vi "TDM Registry.vi"(8 "Details":T2, 9 "Delivery Notifier":refnum<notifier>, 10 "TDM ID":string, 11 "Action":T1) -> (0 "Details out":T2, 1 "Delivery Notifier":refnum<notifier>, 2 "TDM ID out":string, 3 "Found":bool, 4 "TDM Alias Out":string)   [LabVIEW 2020, in "Actor Framework.lvlib"]
uses:
  Actor Framework.lvlib
  Time-Delayed Send Message/Time-Delay Override Options.ctl
  TDM Registration Mode.ctl
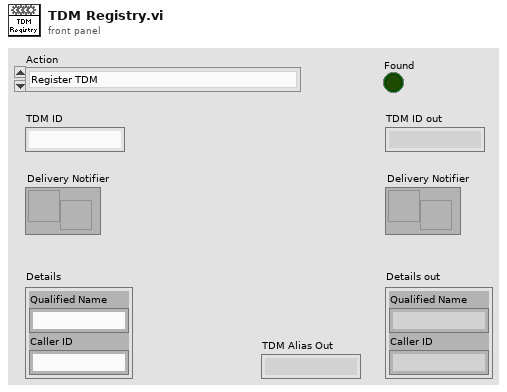
[diagram p1: front panel]
types:
  T1 = typedef "Actor Framework.lvlib/TDM Registration Mode.ctl" = enum16{"Register TDM", "Get ID", "Get Notifier", "Deregister TDM"}
  T2 = cluster{"Qualified Name":string, "Caller ID":string}
  T3 = cluster{"Enqueuers":refnum<notifier>[], "IDs":string[], "Details":cluster{"Qualified Name":string, "Caller ID":string}[]}
  T4 = cluster{"Qualified Name":string, "Caller ID":string}[]
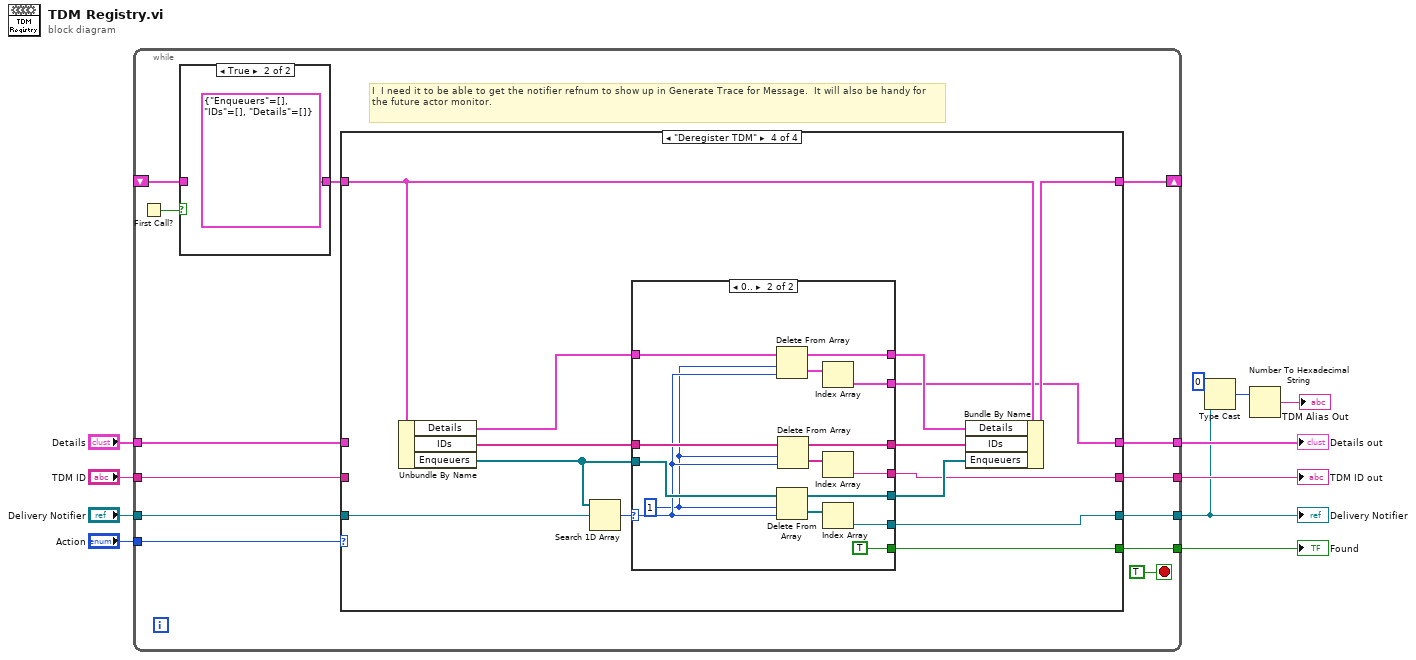
[diagram p0: block diagram]
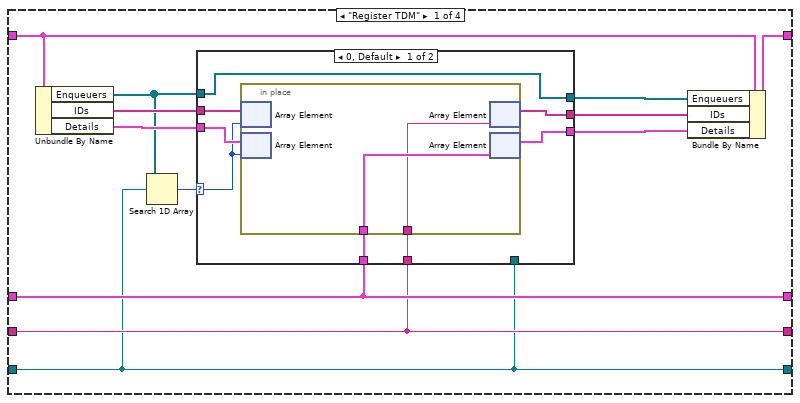
[diagram p3: hidden frame]
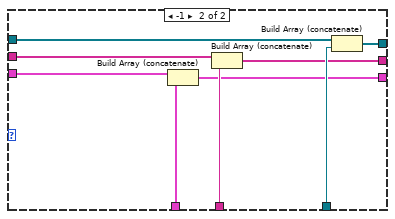
[diagram p4: hidden frame]
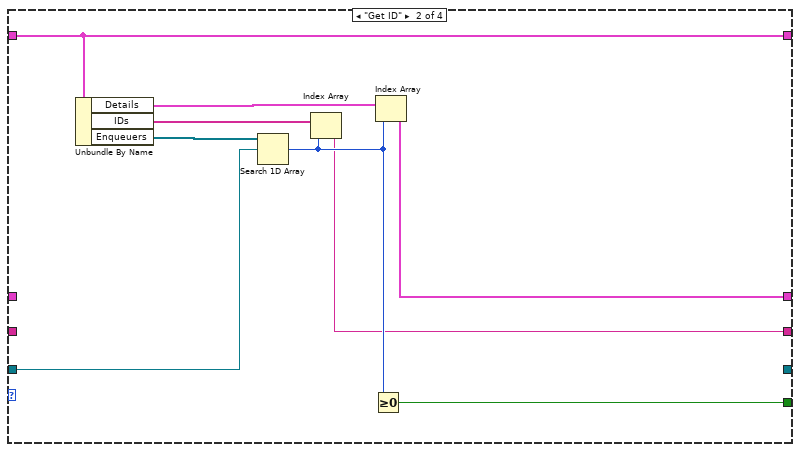
[diagram p5: hidden frame]
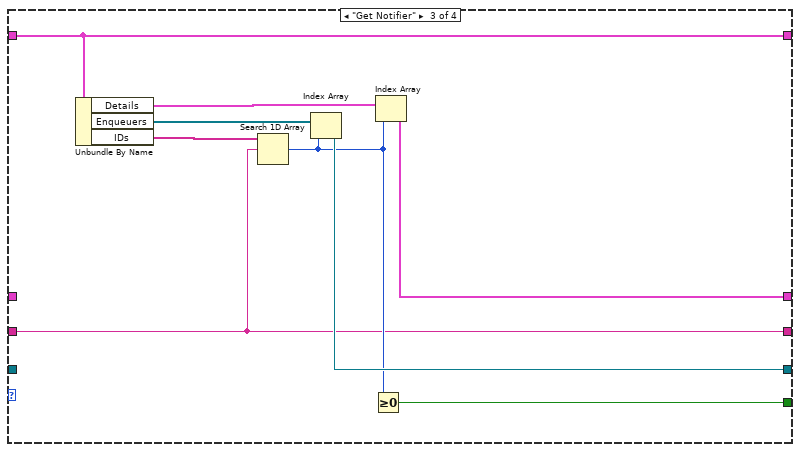
[diagram p6: hidden frame]
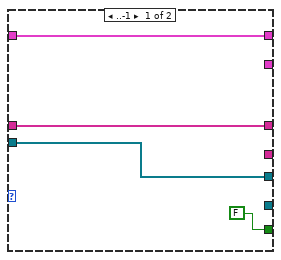
[diagram p7: hidden frame]
diagram:
  n1 = while {
    tunnel: "Action" -> [w24]
    shift-right: [w23] -> _
    shift-left: _ -> [w13]
    tunnel: "TDM ID" -> [w22]
    tunnel: "Delivery Notifier" -> [w21]
    tunnel: "Details" -> [w20]
    tunnel: [w15] -> w5
    tunnel: [w18] -> w7
    tunnel: [w17] -> w6
    tunnel: [w16] -> w2
    stop <- TRUE stop-if-true
    # "I  I need it to be able to get the notifier refnum to show up in Generate Trace for Message.  It will also be handy for the future actor monitor."
    n2 = First Call?() -> (First Call?: T/F=w12:bool)
    n3 = case shown="True" w12 {
      tunnel: [w25 T3 {"Enqueuers"=[], "IDs"=[], "Details"=[]}] -> w14
      tunnel: w13 -> [w25 _]
      frame False {
      }
      frame True {
      }
    }
    n4 = case shown="\"Deregister TDM\"" w24 {
      tunnel: w14 -> [w32 w62 w72 w84]
      tunnel: [w38 w62 w72 w79] -> w23
      tunnel: w22 -> [w28 _ w67 _]
      tunnel: w21 -> [w27 w65 _ w85]
      tunnel: w20 -> [w29 _ _ _]
      tunnel: [w28 w58 w67 w77] -> w15
      tunnel: [w29 w60 w69 w76] -> w18
      tunnel: [_ w61 w71 w80] -> w17
      tunnel: [w27 _ w70 w78] -> w16
      frame "Register TDM" {
        n5 = Unbundle By Name(w32) -> ("Enqueuers"=w31:refnum<notifier>[], "IDs"=w35:string[], "Details"=w34:T4)
        n6 = Search 1D Array(1D array=w31, element=w27) -> (index of element=w30:i32)  [unwired: 1 in]
        n7 = case shown="0, Default" w30 {
          selector: w30 -> [w39 _]
          tunnel: w28 -> [w44 w57]
          tunnel: w27 -> [_ w56]
          tunnel: w29 -> [w45 w55]
          tunnel: w31 -> [w46 w54]
          tunnel: [w46 w53] -> w37
          tunnel: [w41 w52] -> w36
          tunnel: w35 -> [w43 w51]
          tunnel: w34 -> [w42 w50]
          tunnel: [w40 w49] -> w33
          frame 0, Default {
            n8 = in-place {
              in-place-border: w45 -> [w48]
              in-place-border: w44 -> [w47]
              n9 = in-place-array #1(w43, w39) -> ()  [unwired: 1 out]
              n10 = in-place-array #2(w42, w39) -> ()  [unwired: 1 out]
              n11 = in-place-array #1(w47) -> (w41:string[])  [unwired: 1 out]
              n12 = in-place-array #2(w48) -> (w40:T4)  [unwired: 1 out]
            }
          }
          frame -1 {
            n13 = Build Array (concatenate)(w50, w55) -> (w49:T4)
            n14 = Build Array (concatenate)(w51, w57) -> (w52:string[])
            n15 = Build Array (concatenate)(w54, w56) -> (w53:refnum<notifier>[])
          }
        }
        n16 = Bundle By Name(cluster=w32, "Enqueuers"=w37, "IDs"=w36, "Details"=w33) -> (w38:T3)
      }
      frame "Get ID" {
        n17 = Unbundle By Name(w62) -> ("Details"=w64:T4, "IDs"=w63:string[], "Enqueuers"=w66:refnum<notifier>[])
        n18 = Search 1D Array(1D array=w66, element=w65) -> (index of element=w59:i32)  [unwired: 1 in]
        n19 = Index Array(array=w63, index=w59) -> (element=w58:string)
        n20 = Greater Or Equal To 0?(x=w59) -> (x >= 0?=w61:bool)
        n21 = Index Array(array=w64, index=w59) -> (element=w60:T2)
      }
      frame "Get Notifier" {
        n22 = Unbundle By Name(w72) -> ("Details"=w74:T4, "Enqueuers"=w73:refnum<notifier>[], "IDs"=w75:string[])
        n23 = Search 1D Array(1D array=w75, element=w67) -> (index of element=w68:i32)  [unwired: 1 in]
        n24 = Index Array(array=w73, index=w68) -> (element=w70:refnum<notifier>)
        n25 = Greater Or Equal To 0?(x=w68) -> (x >= 0?=w71:bool)
        n26 = Index Array(array=w74, index=w68) -> (element=w69:T2)
      }
      frame "Deregister TDM" {
        n27 = Unbundle By Name(w84) -> ("Details"=w87:T4, "IDs"=w86:string[], "Enqueuers"=w88:refnum<notifier>[])
        n28 = Search 1D Array(1D array=w88, element=w85) -> (index of element=w89:i32)  [unwired: 1 in]
        n29 = case shown="0.." w89 {
          selector: w89 -> [_ w95]
          tunnel: [w91 w108] -> w82
          tunnel: w88 -> [w92 w107]
          tunnel: [w92 w106] -> w83
          tunnel: w86 -> [w91 w105]
          tunnel: [FALSE TRUE] -> w80
          tunnel: w87 -> [w90 w103]
          tunnel: [w90 w102] -> w81
          tunnel: [_ w98] -> w78
          tunnel: [_ w97] -> w77
          tunnel: [_ w96] -> w76
          frame ..-1 {
          }
          frame 0.. {
            w94 = 1 ("length")
            n30 = Delete From Array(array=w103, length=w94, index=w95) -> (deleted portion=w101:T4, array with subset deleted=w102:T4)
            n31 = Delete From Array(array=w107, length=w94, index=w95) -> (deleted portion=w99:refnum<notifier>[], array with subset deleted=w106:refnum<notifier>[])
            n32 = Delete From Array(array=w105, length=w94, index=w95) -> (deleted portion=w100:string[], array with subset deleted=w108:string[])
            n33 = Index Array(array=w101) -> (element=w96:T2)  [unwired: 1 in]
            n34 = Index Array(array=w100) -> (element=w97:string)  [unwired: 1 in]
            n35 = Index Array(array=w99) -> (element=w98:refnum<notifier>)  [unwired: 1 in]
          }
        }
        n36 = Bundle By Name(cluster=w84, "Details"=w81, "IDs"=w82, "Enqueuers"=w83) -> (w79:T3)
      }
    }
  }
  "Delivery Notifier" <- w2
  "TDM ID out" <- w5
  "Details out" <- w7
  "Found" <- w6
  n37 = Type Cast(type=u32 0, x=w2) -> (*(type *) &x=w3:u32)
  n38 = Number To Hexadecimal String(2:w3) -> (0:→"TDM Alias Out":string)  [unwired: 1 in]
